vi "ShutOffSources.vi"(2 "Debug Mode":bool, 3 "Elapsed Time(s)":dbl, 4 "State":enum16{"Edit", "Start", "Run", "End", "Idle"}(ring), 5 "Argument List In":string[](array[string])) -> (0 "Status Out":string, 1 "Argument List Out":string[](array[string]))   [LabVIEW 2011]
panel:
  out "total time":dbl
  out "is OK?":bool
  in  "OK":bool
  out "tTotal(s) 2":dbl
  # "Sources will be shut off"
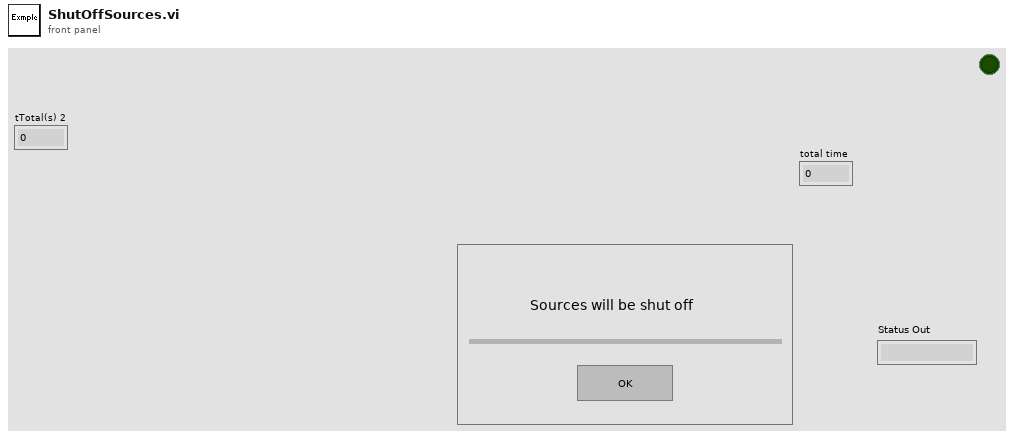
[diagram p1: front panel]
types:
  T1 = enum16{"Discrete", "Continuous", "Instantaneous", "Finite"}
  T2 = enum32{"Invalid", "Default", "Floating", "Floating/Auto-Hide", "Modal"}
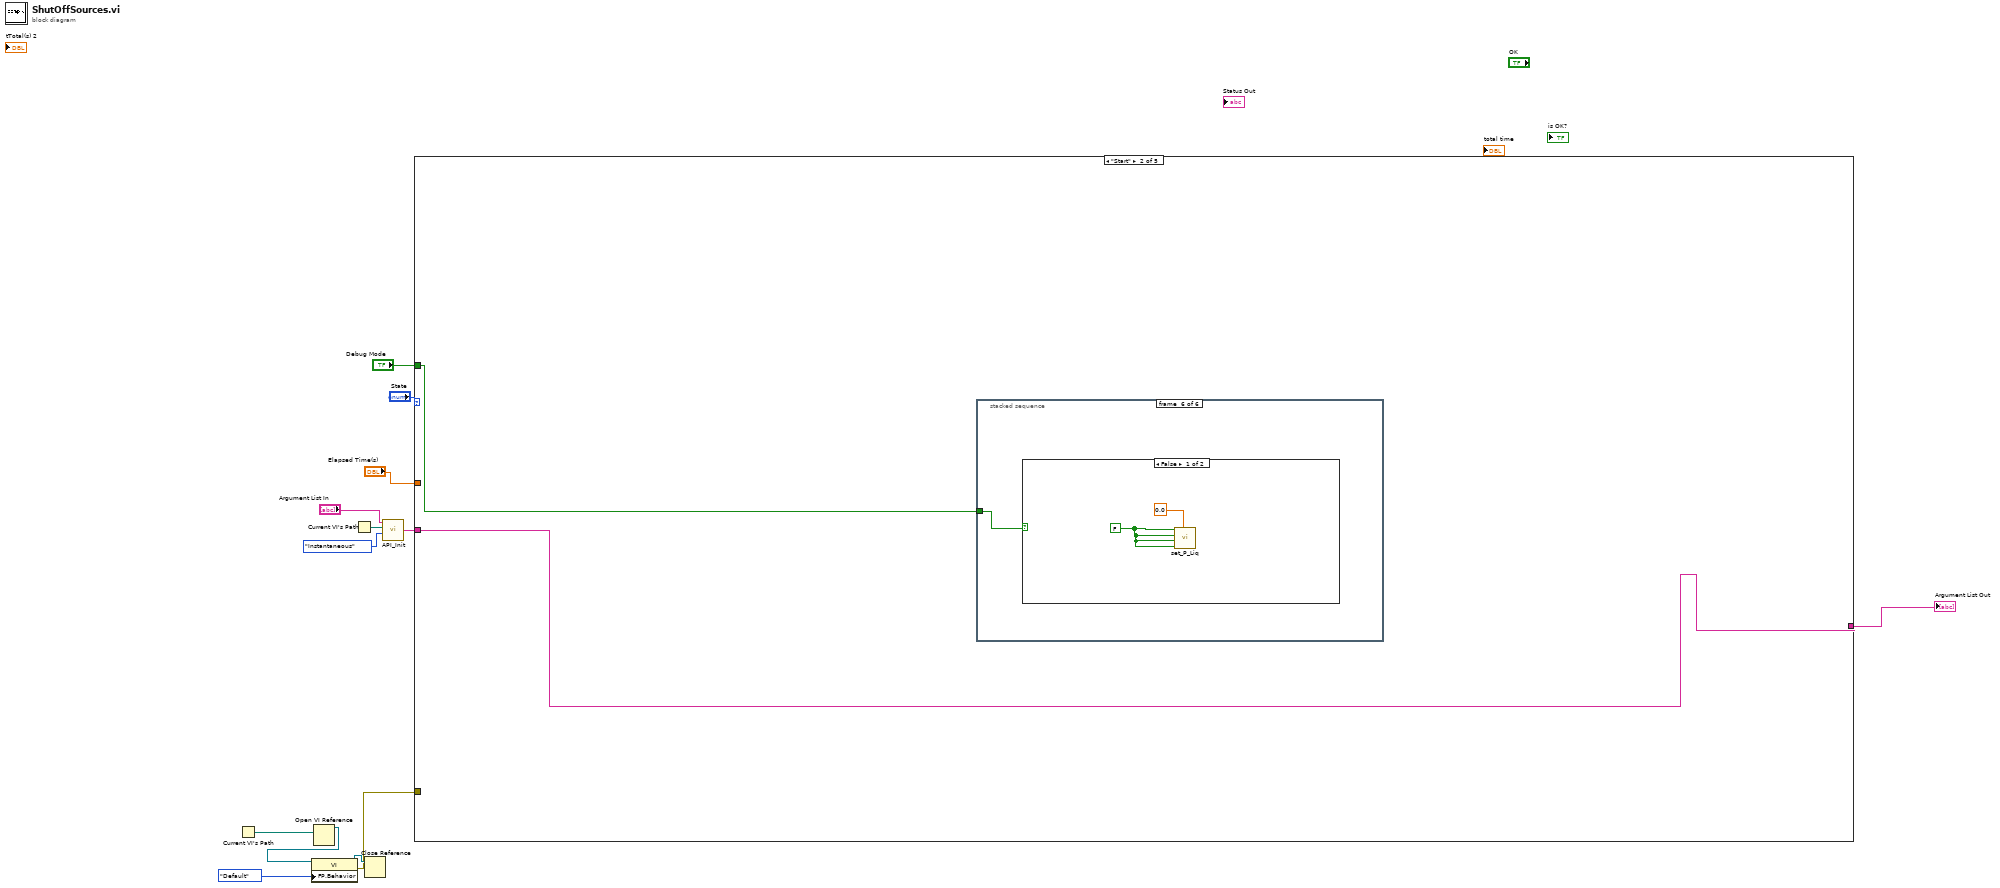
[diagram p0: block diagram]
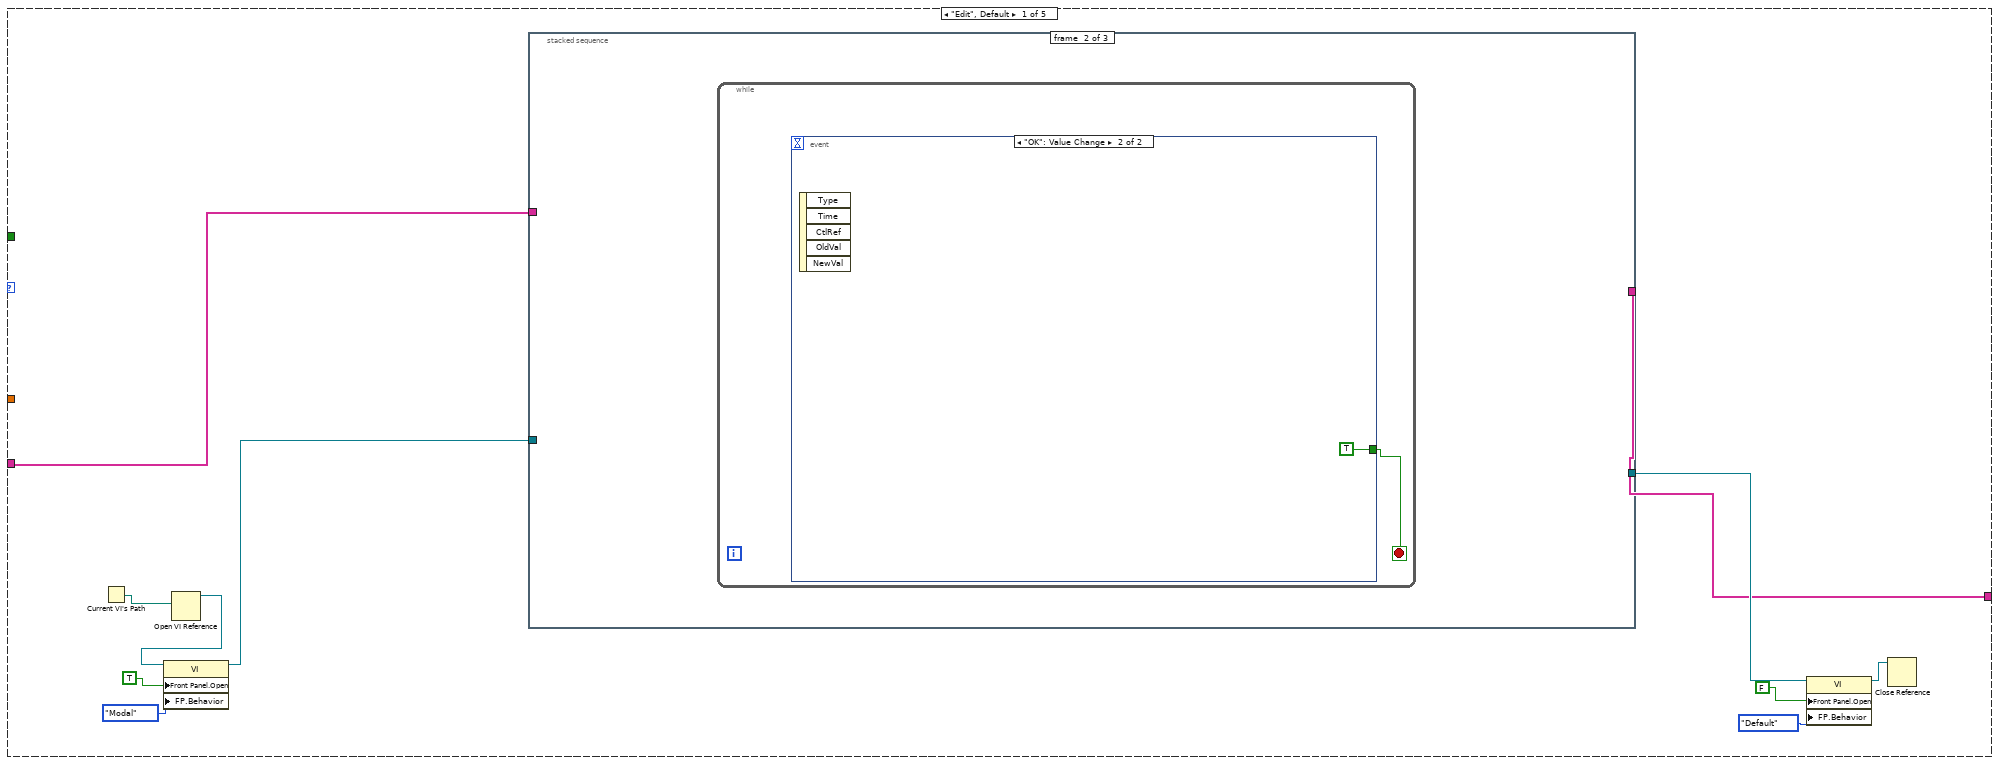
[diagram p2: hidden frame]
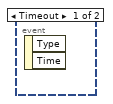
[diagram p4: hidden frame]
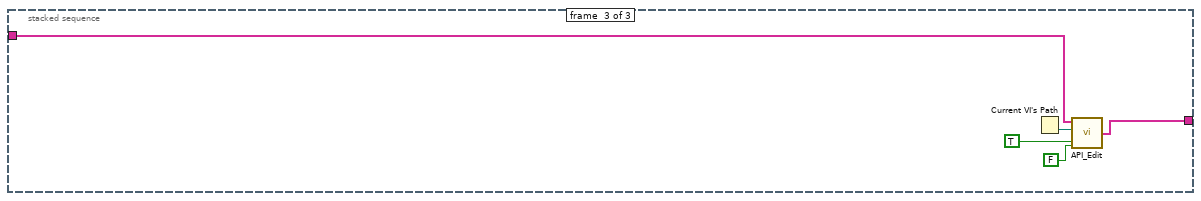
[diagram p5: hidden frame]
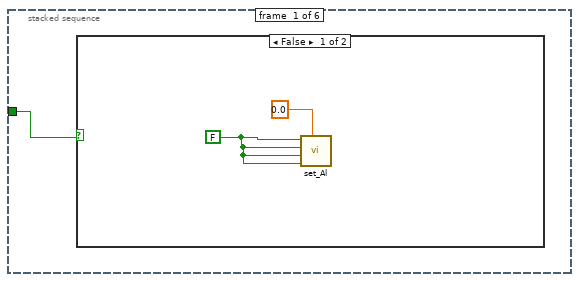
[diagram p6: hidden frame]
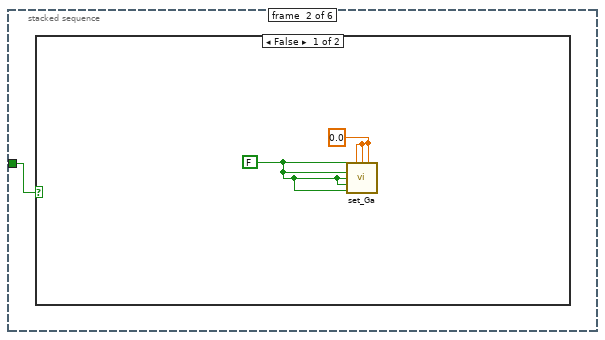
[diagram p8: hidden frame]
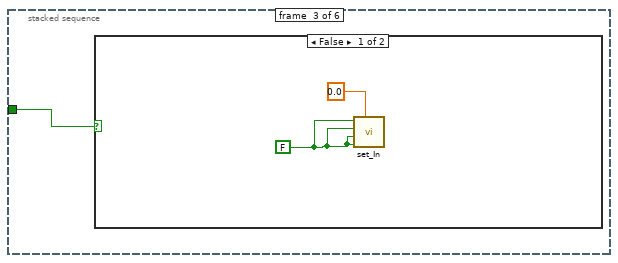
[diagram p10: hidden frame]
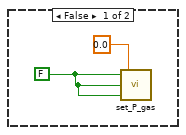
[diagram p13: hidden frame]
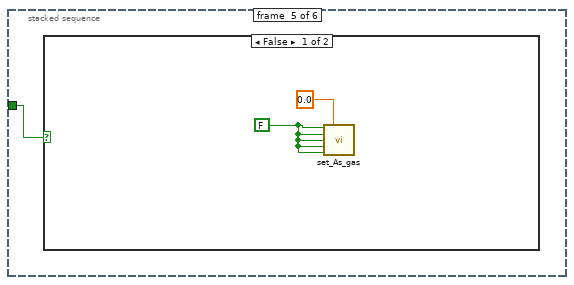
[diagram p14: hidden frame]
diagram:
  n1 = Current VI's Path() -> (path=w9:path)
  n2 = Open VI Reference(vi path=w9) -> (vi reference=w8:refnum<vi>)  [unwired: 1 in, 5 out]
  n3 = property class="VI"(reference=w8, "FP.Behavior"=T2."Default" ("Front Panel Window:Behavior")) -> (reference out=w6:refnum<vi>, error out=w5:errorcluster)  [unwired: 1 in]
  n4 = Current VI's Path() -> (path=w4:path)
  n5 = Close Reference(reference=w6) -> ()  [unwired: 1 in, 1 out]
  n6 = call "API_Init.vi"("API Mode"=T1."Instantaneous", "VI Path"=w4, "Argument List In"="Argument List In") -> ("Argument List Out"=w1:string[])  [unwired: 1 in]
  n7 = case shown="\"Start\"" "State" {
    tunnel: "Debug Mode" -> [_ w33 _ _ _]
    tunnel: "Elapsed Time(s)" -> [_ _ _ _ _]
    tunnel: w1 -> [w15 w34 w53 w54 w55]
    tunnel: [w14 w34 w53 w54 w55] -> w10
    tunnel: w5 -> [_ _ _ _ _]
    frame "Edit", Default {
      n8 = Current VI's Path() -> (path=w20:path)
      n9 = Open VI Reference(vi path=w20) -> (vi reference=w19:refnum<vi>)  [unwired: 1 in, 5 out]
      n10 = property class="VI"(reference=w19, "Front Panel.Open"=TRUE ("Front Panel Window:Open"), "FP.Behavior"=T2."Modal" ("Front Panel Window:Behavior")) -> (reference out=w18:refnum<vi>)  [unwired: 1 in, 1 out]
      n11 = stacked-sequence {
        tunnel: w15 -> [_ _ w30]
        tunnel: w18 -> [w25 _ _]
        tunnel: [w25 _ _] -> w22
        tunnel: [_ _ w31] -> w14
        frame #0 {
        }
        frame #1 {
          n12 = while {
            stop <- w26 stop-if-true
            n13 = event shown="[1] \"OK\": Value Change" {
              selector: _ -> [_ _]
              dyn-events: _ -> [_ _]
              timeout: _ -> [_ _]
              tunnel: [_ TRUE] -> w26
              event Timeout {
                n14 = event-data() -> ()  [unwired: 1 in, 2 out]
              }
              event "OK": Value Change {
                n15 = event-data() -> ()  [unwired: 1 in, 5 out]
              }
            }
          }
        }
        frame #2 {
          n16 = Current VI's Path() -> (path=w32:path)
          n17 = call "API_Edit.vi"("Cancel"=FALSE, "OK"=TRUE, "VI Path"=w32, "Argument List In"=w30) -> ("Argument List Out"=w31:string[])
        }
      }
      n18 = property class="VI"(reference=w22, "Front Panel.Open"=FALSE ("Front Panel Window:Open"), "FP.Behavior"=T2."Default" ("Front Panel Window:Behavior")) -> (reference out=w23:refnum<vi>)  [unwired: 1 in, 1 out]
      n19 = Close Reference(reference=w23) -> ()  [unwired: 1 in, 1 out]
    }
    frame "Start" {
      n20 = stacked-sequence {
        tunnel: w33 -> [w35 w38 w41 w44 w47 w50]
        frame #0 {
          n21 = case shown="False" w35 {
            frame False {
              w37 = FALSE ("Al Active")
              n22 = call "set_Al.vi"("ALMFC1"=0.0 ("Aluminum Flow"), "Remote"=w37, "Run"=w37, "Bubbler In"=w37, "Active"=w37) -> ()  [unwired: 5 out]
            }
            frame True {
            }
          }
        }
        frame #1 {
          n23 = case shown="False" w38 {
            frame False {
              w40 = FALSE ("Ga Active")
              w39 = 0.0 ("Ga Flow 1")
              n24 = call "set_Ga.vi"("Active"=w40, "GAMFC3"=w39, "GAMFC2"=w39, "GAMFC1"=w39, "Bubbler In"=w40, "H2 Dilute"=w40, "Run"=w40, "Remote"=w40) -> ()  [unwired: 8 out]
            }
            frame True {
            }
          }
        }
        frame #2 {
          n25 = case shown="False" w41 {
            frame False {
              w43 = FALSE ("In Remote")
              n26 = call "set_In.vi"("INMFC1"=0.0 ("Indium Flow"), "Remote"=w43, "Run"=w43, "Bubbler In"=w43, "Active"=w43) -> ()  [unwired: 5 out]
            }
            frame True {
            }
          }
        }
        frame #3 {
          n27 = case shown="True" w44 {
            frame False {
              w45 = FALSE ("P_Gas Active")
              n28 = call "set_P_gas.vi"("Run"=w45, "Gas In"=w45, "Active"=w45, "P_Gas Remote"=w45, "H2 Flush"=w45, "P_Gas Flow"=0.0) -> ()
            }
            frame True {
            }
          }
        }
        frame #4 {
          n29 = case shown="False" w47 {
            frame False {
              w48 = FALSE ("As_Gas Active")
              n30 = call "set_As_gas.vi"("Active"=w48, "As_Gas Flow"=0.0, "Gas In"=w48, "H2 Flush"=w48, "Run"=w48, "Remote"=w48) -> ()  [unwired: 10 in]
            }
            frame True {
            }
          }
        }
        frame #5 {
          n31 = case shown="False" w50 {
            frame False {
              w52 = FALSE ("Al Active")
              n32 = call "set_P_Liq.vi"("INMFC1"=0.0 ("Aluminum Flow"), "Remote"=w52, "Run"=w52, "Bubbler In"=w52, "Active"=w52) -> ()  [unwired: 5 in]
            }
            frame True {
            }
          }
        }
      }
    }
    frame "Run" {
    }
    frame "End" {
    }
    frame "Idle" {
    }
  }
  "Argument List Out" <- w10
